vi "Source Panel.vi"(8 "error in":errorcluster, 11 "src in":T1={"type"=enum."Tektronix AFG3101C", "afg"={"VISA"="", "const"=0.0, "gen DC"=FALSE, "ext ref"=FALSE}, "cDAQ dds"={"device"="", "channels"=[], "mclk source"="", "mclk [Hz]"=0.0, "fs [Hz]"=0.0, "block [s]"=0.0, "buf [s]"=0.0, "task"="", "cmd queue"=refnum, "proc ref"=refnum, "smpl clock out"="/cDAQ3/PFI0", "export smpl clock"=FALSE, "DC ofs [V]"=[], "timebase source"="", "timebase mode"=enum."Local", "dither"=enum."Disabled", "dither level"=0.0, "phase [rad]"=[]}, "gain [V/A]"=1.0, "F5xxx session"={"VISA"="", "mode"=enum."AC voltage", "Earth on"=FALSE, "Ext ref lock"=FALSE}, "t3awg"={"VISA"="", "use ext ref"=FALSE, "ext ref [Hz]"=0.0, "load Z"=enum."High Z", "ramdac max n"=0, "noise dither [V]"=0.0, "t3awg fs rules"=[], "channels"=0, "ramdac min n"=0}} {"t3awg"."t3awg fs rules"."fs-step [Hz]" format="%#_6p"; "t3awg"."t3awg fs rules"."fs-max [Hz]" format="%#_6p"; "t3awg"."t3awg fs rules"."for f0 <" format="%#_6p"; "t3awg"."t3awg fs rules"."fs-min [Hz]" format="%#_6p"; "cDAQ dds"."channels" min=0 step=1}) -> (0 "error out":errorcluster, 3 "src out":T1={"type"=enum."Tektronix AFG3101C", "afg"={"VISA"="", "const"=0.0, "gen DC"=FALSE, "ext ref"=FALSE}, "cDAQ dds"={"device"="", "channels"=[], "mclk source"="", "mclk [Hz]"=0.0, "fs [Hz]"=0.0, "block [s]"=0.0, "buf [s]"=0.0, "task"="", "cmd queue"=refnum, "proc ref"=refnum, "smpl clock out"="/cDAQ3/PFI0", "export smpl clock"=FALSE, "DC ofs [V]"=[], "timebase source"="", "timebase mode"=enum."Local", "dither"=enum."Disabled", "dither level"=0.0, "phase [rad]"=[]}, "gain [V/A]"=1.0, "F5xxx session"={"VISA"="", "mode"=enum."AC voltage", "Earth on"=FALSE, "Ext ref lock"=FALSE}, "t3awg"={"VISA"="", "use ext ref"=FALSE, "ext ref [Hz]"=0.0, "load Z"=enum."High Z", "ramdac max n"=0, "noise dither [V]"=0.0, "t3awg fs rules"=[], "channels"=0, "ramdac min n"=0}} {"t3awg"."t3awg fs rules"."fs-step [Hz]" format="%#_6p"; "t3awg"."t3awg fs rules"."fs-max [Hz]" format="%#_6p"; "t3awg"."t3awg fs rules"."for f0 <" format="%#_6p"; "t3awg"."t3awg fs rules"."fs-min [Hz]" format="%#_6p"; "cDAQ dds"."channels" min=0 step=1})   [LabVIEW 2020]
uses:
  Source Type.ctl
  Source Session.ctl
  drivers/AFG3101C/AFG3101C Session.ctl
  drivers/cDAQ DDS/cDAQ DDS Session.ctl
  drivers/cDAQ DDS/cDAQ DDS Setup.ctl
  drivers/cDAQ DDS/cDAQ DDS Timebase Mode.ctl
  drivers/cDAQ DDS/cDAQ DDS Dither.ctl
  drivers/Fluke 5XXX/top_lev/F5xxx_session.ctl
  drivers/Fluke 5XXX/top_lev/F5xxx_output_mode.ctl
  drivers/T3AWG3K/toplevel/T3AWG Session.ctl
  drivers/T3AWG3K/toplevel/T3AWG Load Z.ctl
  drivers/T3AWG3K/toplevel/fgen_ramdac_fs_rules.ctl
  drivers/T3AWG3K/Active Technologies AWG3000.lvlib
panel:
  in  "btn default":bool
  in  "tc src 2":enum32{"dummy"}(tab)
  in  "afg gain":dbl caption="Amplifier gain constant [V/A]" format="%0_6g"
  in  "btn cancel":bool
  in  "btn ok":bool
  in  "type":T2 caption="Generator type"
  in  "tc src":T12(tab)
  in  "afg ext ref":bool caption="External reference clock"
  in  "afg visa":refnum<visa-resource-name> caption="VISA address"
  in  "afg gen dc":bool caption="Generate DC bias"
  in  "btn cfg cdaq":bool
  in  "btn cfg fluke":bool
  in  "btn cfg t3awg":bool
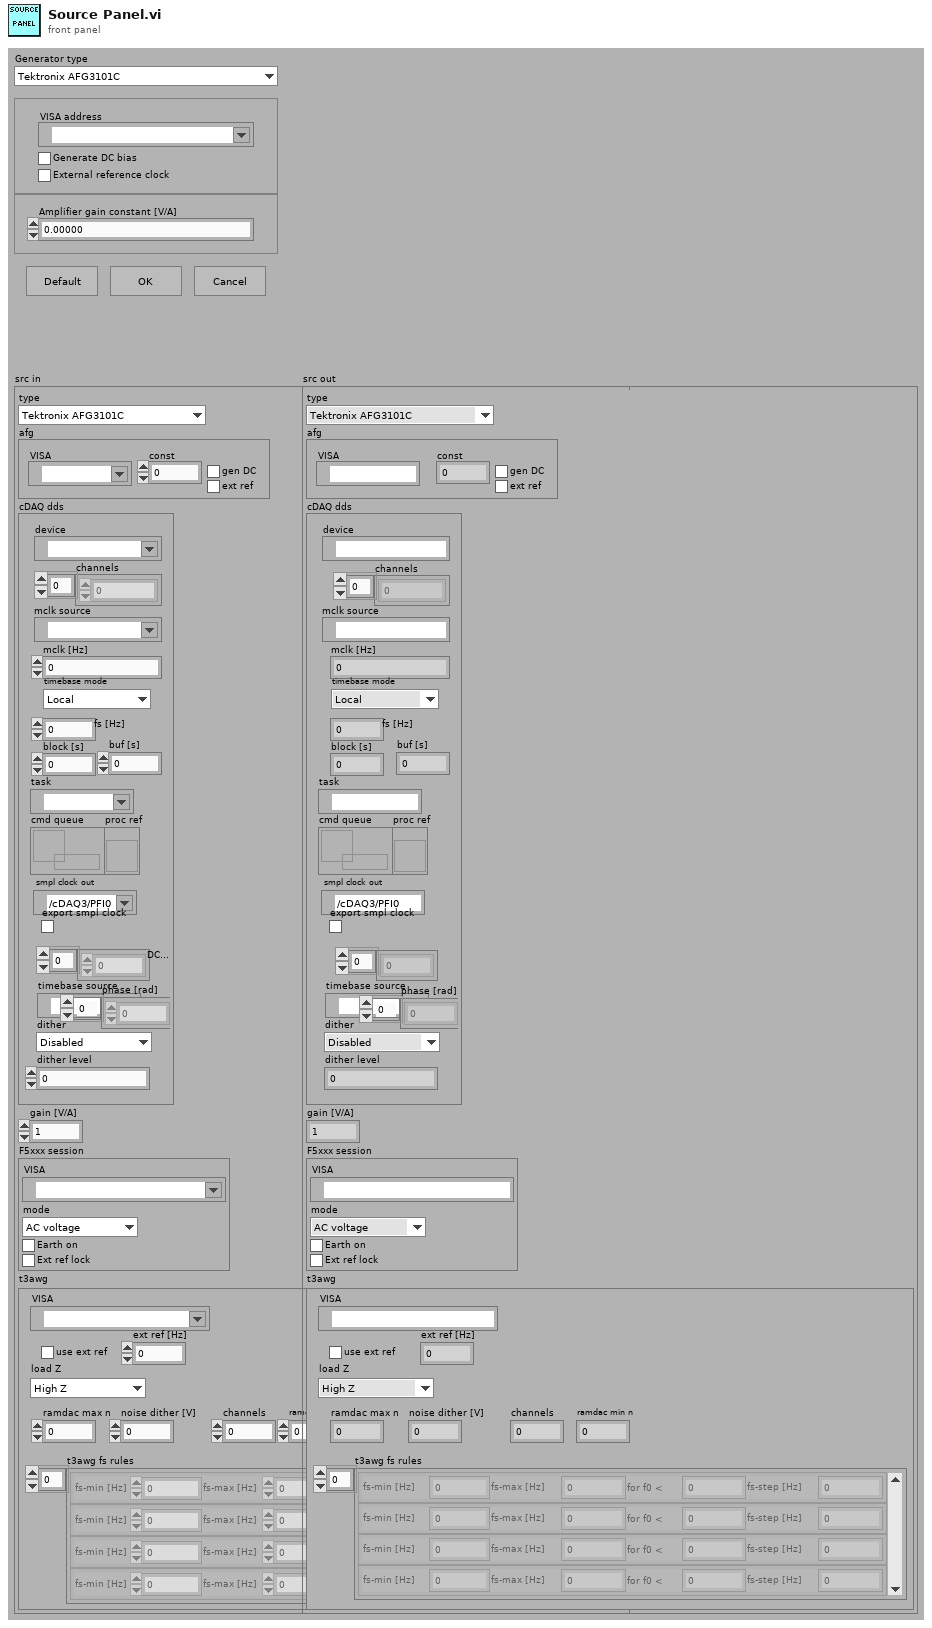
[diagram p1: front panel]
types:
  T1 = typedef "Source Session.ctl" = cluster{"type":T2, "afg":T3, "cDAQ dds":T4, "gain [V/A]":dbl, "F5xxx session":T7, "t3awg":T9}
  T2 = typedef "Source Type.ctl" = enum16{"Tektronix AFG3101C", "cDAQ DAC", "Fluke 5xxx", "Agilent 33120A", "R&S SMT", "Teledyne LeCroy T3AWG", "dummy"}
  T3 = typedef "AFG3101C Session.ctl" = cluster{"VISA":refnum<visa-resource-name>, "const":dbl, "gen DC":bool, "ext ref":bool}
  T4 = typedef "cDAQ DDS Session.ctl" = cluster{"device":tag, "channels":i32[], "mclk source":tag, "mclk [Hz]":dbl, "fs [Hz]":dbl, "block [s]":dbl, "buf [s]":dbl, "task":refnum<k21>, "cmd queue":refnum<queue>, "proc ref":refnum<vi>, "smpl clock out":tag, "export smpl clock":bool, "DC ofs [V]":dbl[], "timebase source":tag, "timebase mode":T5, "dither":T6, "dither level":dbl, "phase [rad]":dbl[]}
  T5 = typedef "cDAQ DDS Timebase Mode.ctl" = enum16{"Local", "Take from ADC (e.g. NI 9238)", "Other source"}
  T6 = typedef "cDAQ DDS Dither.ctl" = enum16{"Disabled", "Gaussian"}
  T7 = typedef "F5xxx_session.ctl" = cluster{"VISA":refnum<visa-resource-name>, "mode":T8, "Earth on":bool, "Ext ref lock":bool}
  T8 = typedef "F5xxx_output_mode.ctl" = enum16{"AC voltage", "AC current"}
  T9 = typedef "Active Technologies AWG3000.lvlib/T3AWG Session.ctl" = cluster{"VISA":refnum<visa-resource-name>, "use ext ref":bool, "ext ref [Hz]":dbl, "load Z":T10, "ramdac max n":i32, "noise dither [V]":dbl, "t3awg fs rules":T11[], "channels":i32, "ramdac min n":i32}
  T10 = typedef "Active Technologies AWG3000.lvlib/T3AWG Load Z.ctl" = enum16{"High Z", "50 Ohm"}
  T11 = typedef "Active Technologies AWG3000.lvlib/fgen_ramdac_fs_rules.ctl" = cluster{"fs-min [Hz]":dbl, "fs-max [Hz]":dbl, "for f0 < ":dbl, "fs-step [Hz]":dbl}
  T12 = enum32{"AWG", "cDAQ DDS", "F5xxx", "T3AWG", "dummy"}
  T13 = enum32{"AWG", "cDAQ DDS", "F5xxx", "T3AWG", "dummy"}[]
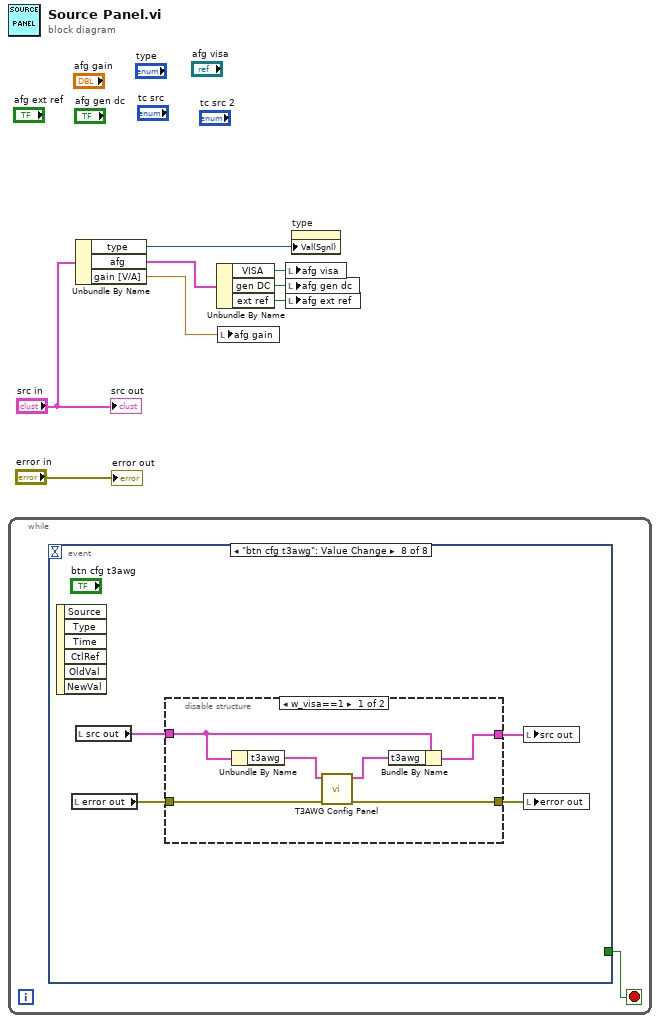
[diagram p0: block diagram]
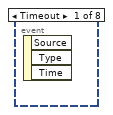
[diagram p2: hidden frame]
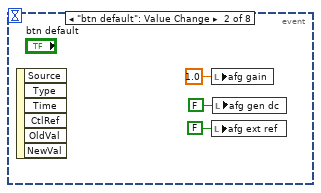
[diagram p3: hidden frame]
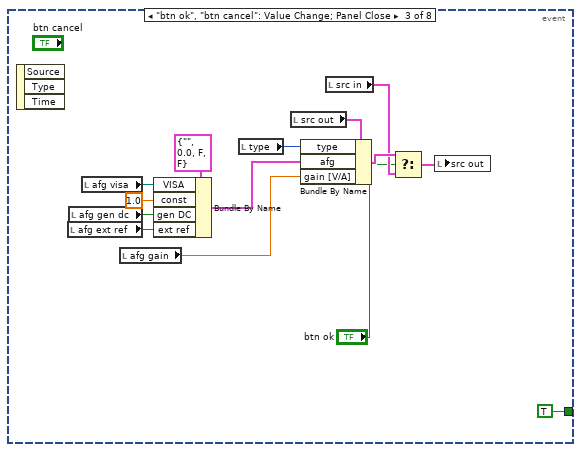
[diagram p4: hidden frame]
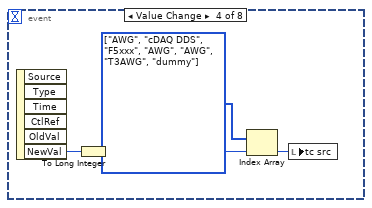
[diagram p5: hidden frame]
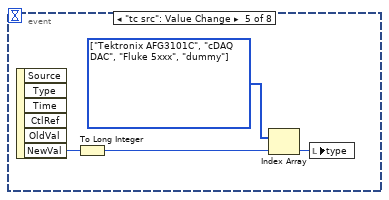
[diagram p6: hidden frame]
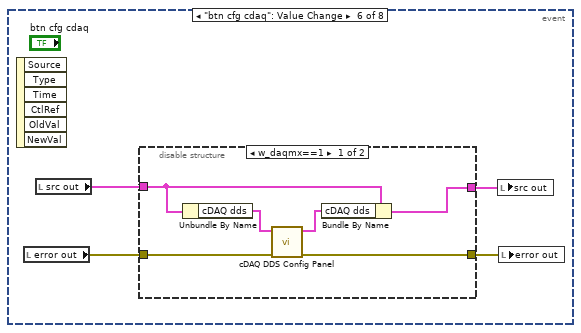
[diagram p7: hidden frame]
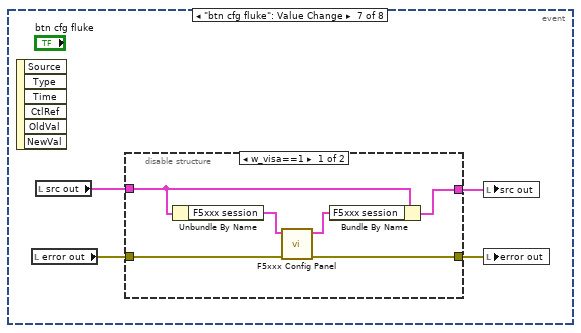
[diagram p9: hidden frame]
diagram:
  n1 = while {
    stop <- w9 stop-if-true
    n2 = event shown="[7] \"btn cfg t3awg\": Value Change" {
      selector: _ -> [_ _ _ _ _ _ _ _]
      dyn-events: _ -> [_ _ _ _ _ _ _ _]
      timeout: _ -> [_ _ _ _ _ _ _ _]
      tunnel: [_ _ TRUE _ _ _ _ _] -> w9
      event Timeout {
        n3 = event-data() -> ()  [unwired: 1 in, 3 out]
      }
      event "btn default": Value Change {
        n4 = event-data() -> ()  [unwired: 1 in, 6 out]
        n5 = local write "afg gain"(1.0 ("afg gain")) -> ()
        n6 = local write "afg ext ref"(FALSE ("afg ext ref")) -> ()
        n7 = local write "afg gen dc"(FALSE ("afg gen dc")) -> ()
      }
      event "btn ok", "btn cancel": Value Change; Panel Close {
        n8 = event-data() -> ()  [unwired: 1 in, 3 out]
        n9 = local read "afg ext ref"() -> (w13:bool)
        n10 = local read "afg gen dc"() -> (w22:bool)
        n11 = local read "afg visa"() -> (w23:refnum<visa-resource-name>)
        n12 = local read "afg gain"() -> (w15:dbl)
        n13 = Bundle By Name(cluster=T3 {"VISA"="", "const"=0.0, "gen DC"=FALSE, "ext ref"=FALSE} ("afg"), "VISA"=w23, "const"=1.0, "gen DC"=w22, "ext ref"=w13) -> (w21:T3)
        n14 = local read "type"() -> (w25:T2)
        n15 = local read "src out"() -> (w14:T1)
        n16 = Bundle By Name(cluster=w14, "type"=w25, "afg"=w21, "gain [V/A]"=w15) -> (w20:T1)
        n17 = local read "src in"() -> (w19:T1)
        n18 = Select(t=w20, s="btn ok", f=w19) -> (s? t:f=w17:T1)
        n19 = local write "src out"(w17) -> ()
      }
      event Value Change {
        w28 = T13 [enum."AWG", enum."cDAQ DDS", enum."F5xxx", enum."AWG", enum."AWG", enum."T3AWG", enum."dummy"] items=["AWG", "cDAQ DDS", "F5xxx", "T3AWG", "dummy"]
        n20 = event-data() -> ("NewVal"=w30:T2)  [unwired: 1 in, 5 out]
        n21 = To Long Integer(number=w30) -> (32bit integer=w29:i32)
        n22 = Index Array(array=w28, index=w29) -> (element=w27:T12)
        n23 = local write "tc src"(w27) -> ()
      }
      event "tc src": Value Change {
        w32 = T2[] [enum."Tektronix AFG3101C", enum."cDAQ DAC", enum."Fluke 5xxx", enum."dummy"] items=["Tektronix AFG3101C", "cDAQ DAC", "Fluke 5xxx", "Agilent 33120A", "R&S SMT", "Teledyne LeCroy T3AWG", "dummy"]
        n24 = event-data() -> ("NewVal"=w34:T12)  [unwired: 1 in, 5 out]
        n25 = To Long Integer(number=w34) -> (32bit integer=w33:i32)
        n26 = Index Array(array=w32, index=w33) -> (element=w31:T2)
        n27 = local write "type"(w31) -> ()
      }
      event "btn cfg cdaq": Value Change {
        n28 = event-data() -> ()  [unwired: 1 in, 6 out]
        n29 = local read "error out"() -> (w38:errorcluster)
        n30 = local read "src out"() -> (w36:T1)
        n31 = disable-structure shown="w_daqmx==1" {
          disable-tunnel: w38 -> [w44 w46]
          disable-tunnel: [w43 w46] -> w37
          disable-tunnel: w36 -> [w41 w45]
          disable-tunnel: [w39 w45] -> w35
          frame condition #0 (active) {
            n32 = Unbundle By Name(w41) -> ("cDAQ dds"=w42:T4)
            n33 = call "cDAQ DDS Config Panel.vi"("error in"=w44, "cDAQ dds"=w42) -> ("error out"=w43:errorcluster, "cDAQ dds out"=w40:T4)  [unwired: 8 in]
            n34 = Bundle By Name(cluster=w41, "cDAQ dds"=w40) -> (w39:T1)
          }
          frame condition #1 {
          }
        }
        n35 = local write "src out"(w35) -> ()
        n36 = local write "error out"(w37) -> ()
      }
      event "btn cfg fluke": Value Change {
        n37 = event-data() -> ()  [unwired: 1 in, 6 out]
        n38 = local read "error out"() -> (w50:errorcluster)
        n39 = local read "src out"() -> (w48:T1)
        n40 = disable-structure shown="w_visa==1" {
          disable-tunnel: w50 -> [w56 w58]
          disable-tunnel: [w55 w58] -> w49
          disable-tunnel: w48 -> [w54 w57]
          disable-tunnel: [w52 w57] -> w47
          frame condition #0 (active) {
            n41 = Unbundle By Name(w54) -> ("F5xxx session"=w51:T7)
            n42 = call "F5xxx Config Panel.vi"("error in"=w56, "session in"=w51) -> ("error out"=w55:errorcluster, "session out"=w53:T7)  [unwired: 8 in]
            n43 = Bundle By Name(cluster=w54, "F5xxx session"=w53) -> (w52:T1)
          }
          frame condition #1 {
          }
        }
        n44 = local write "src out"(w47) -> ()
        n45 = local write "error out"(w49) -> ()
      }
      event "btn cfg t3awg": Value Change {
        n46 = event-data() -> ()  [unwired: 1 in, 6 out]
        n47 = local read "error out"() -> (w62:errorcluster)
        n48 = local read "src out"() -> (w60:T1)
        n49 = disable-structure shown="w_visa==1" {
          disable-tunnel: w62 -> [w68 w70]
          disable-tunnel: [w67 w70] -> w61
          disable-tunnel: w60 -> [w66 w69]
          disable-tunnel: [w64 w69] -> w59
          frame condition #0 (active) {
            n50 = Unbundle By Name(w66) -> ("t3awg"=w63:T9)
            n51 = call "T3AWG Config Panel.vi"("error in (no error)"=w68, "t3awg in"=w63) -> ("error out"=w67:errorcluster, "t3awg out"=w65:T9)  [unwired: 8 in]
            n52 = Bundle By Name(cluster=w66, "t3awg"=w65) -> (w64:T1)
          }
          frame condition #1 {
          }
        }
        n53 = local write "src out"(w59) -> ()
        n54 = local write "error out"(w61) -> ()
      }
    }
  }
  n55 = Unbundle By Name("src in") -> ("type"=w6:T2, "afg"=w5:T3, "gain [V/A]"=w2:dbl)
  n56 = Unbundle By Name(w5) -> ("VISA"=w4:refnum<visa-resource-name>, "gen DC"=w3:bool, "ext ref"=w1:bool)
  n57 = local write "afg gain"(w2) -> ()
  n58 = local write "afg visa"(w4) -> ()
  n59 = local write "afg gen dc"(w3) -> ()
  n60 = local write "afg ext ref"(w1) -> ()
  n61 = property on="type" class="Enum (strict)"("Val(Sgnl)"=w6) -> ()  [unwired: 2 in, 2 out]
  "error out" <- "error in"
  "src out" <- "src in"
